vi "createAVIRefnum.vi"(5 "Video:heigth [px]":i32, 7 "Video:width [px]":i32, 8 "error in":errorcluster, 9 "Video:rotate":bool, 10 "Video file path":path, 11 "Input cluster":T1) -> (0 "error out":errorcluster, 3 "Output cluster":T1)   [LabVIEW 2020]
doc: "Create Refnum from .avi file with given name"
uses:
  controls/StateMachineVariables.ctl
  <vilib>/vision/Avi.llb/IMAQ AVI2 Refnum.ctl
  <vilib>/userDefined/High Color/IMAQdx.ctl
  <vilib>/vision/Deep Learning.llb/IMAQ DL Model Refnum.ctl
  <vilib>/vision/Image Controls.llb/IMAQ Image.ctl
  <vilib>/vision/Avi.llb/IMAQ AVI2 Codec Path.ctl
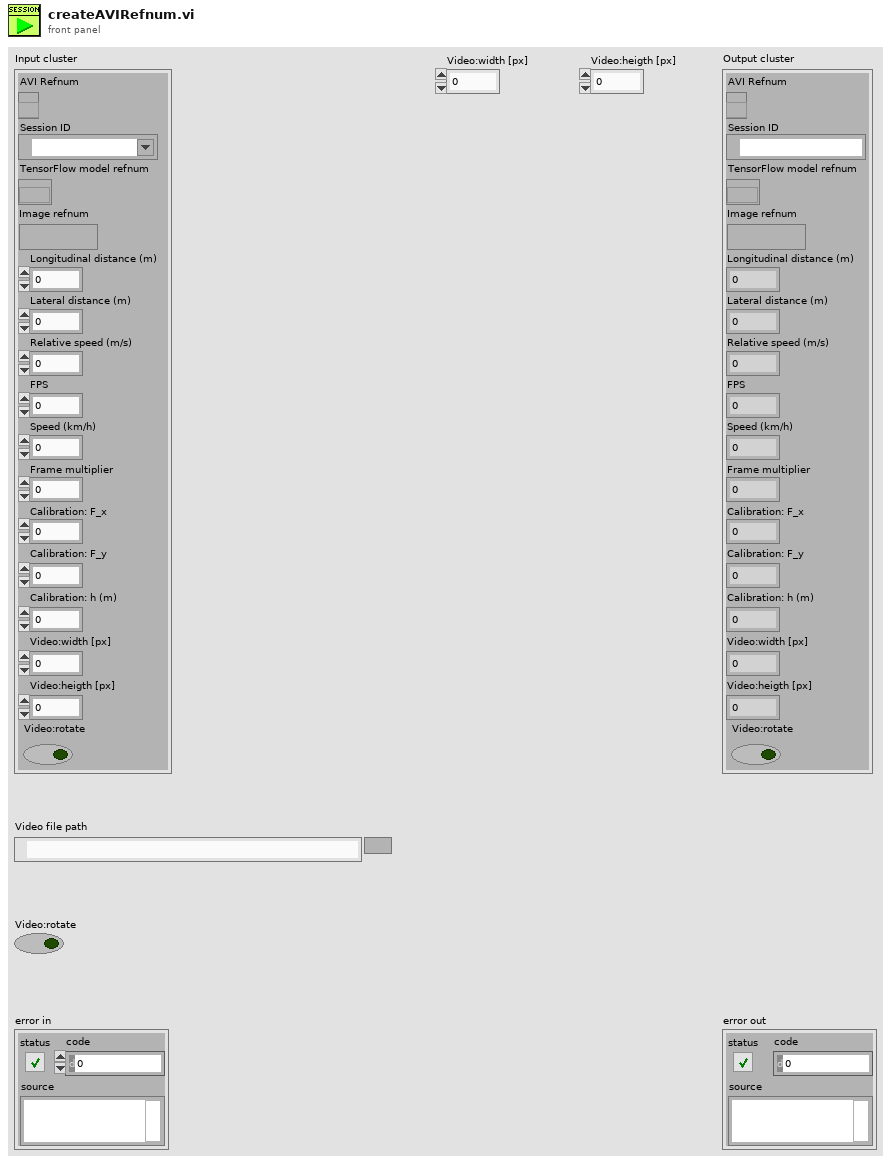
[diagram p1: front panel]
types:
  T1 = typedef "StateMachineVariables.ctl" = cluster{"AVI Refnum":T2, "Session ID":T3, "TensorFlow model refnum":T4, "Image refnum":T5, "Longitudinal distance (m)":dbl, "Lateral distance (m)":dbl, "Relative speed (m/s)":dbl, "FPS":dbl, "Speed (km/h)":dbl, "Frame multiplier":u32, "Calibration: F_x":dbl, "Calibration: F_y":dbl, "Calibration: h (m)":dbl, "Video:width [px]":i32, "Video:heigth [px]":i32, "Video:rotate":bool}
  T2 = typedef "IMAQ AVI2 Refnum.ctl" = refnum<k20>
  T3 = typedef "IMAQdx.ctl" = refnum<k21>
  T4 = typedef "IMAQ DL Model Refnum.ctl" = refnum<k20>
  T5 = typedef "IMAQ Image.ctl" = refnum<image>
  T6 = typedef "IMAQ AVI2 Codec Path.ctl" = u32
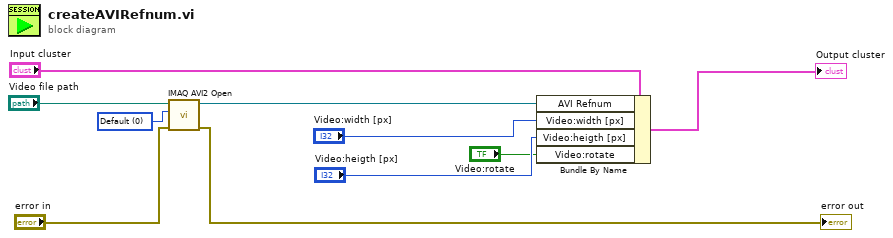
[diagram p0: block diagram]
diagram:
  w2 = T6 0 items=["Default", "System", "Built in Vision"] ("Codec Source")
  n1 = call "IMAQ AVI2 Open"("error in (no error)"="error in", "Codec Source"=w2, "AVI File Path"="Video file path") -> ("error out"=→"error out":errorcluster, "AVI Refnum"=w9:T2)  [unwired: 7 in]
  n2 = Bundle By Name(cluster="Input cluster", "AVI Refnum"=w9, "Video:width [px]"="Video:width [px]", "Video:heigth [px]"="Video:heigth [px]", "Video:rotate"="Video:rotate") -> (→"Output cluster":T1)
